vi "Automatic EMS.vi"(8 "error in":errorcluster, 11 "Master Controller in":refnum<class "EMS User Interface.lvclass">) -> (0 "error out":errorcluster, 3 "dup Master Controller out":refnum<class "EMS User Interface.lvclass">)   [LabVIEW 2018, in "EMS User Interface Actor.lvlib" / "EMS User Interface.lvclass"]
uses:
  EMS User Interface.lvclass
  EMS User Interface.lvclass/EMS User Interface.ctl
  <vilib>/ActorFramework/Message Enqueuer/Message Enqueuer.lvclass/Message Enqueuer.ctl
  <vilib>/ActorFramework/Message Enqueuer/Message Priority.ctl
  <vilib>/ActorFramework/Message Enqueuer/Enqueue.vi
  EMS Core/EMS Messages/Stop Init Msg/Stop Init Msg.lvclass
  C:/Program Files (x86)/National Instruments/LabVIEW 2018/vi.lib/ActorFramework/Message/Message.lvclass
  <vilib>/ActorFramework/Message Priority Queue/Priority Enqueue.vi
  <vilib>/ActorFramework/Message Enqueuer/Message Enqueuer.lvclass
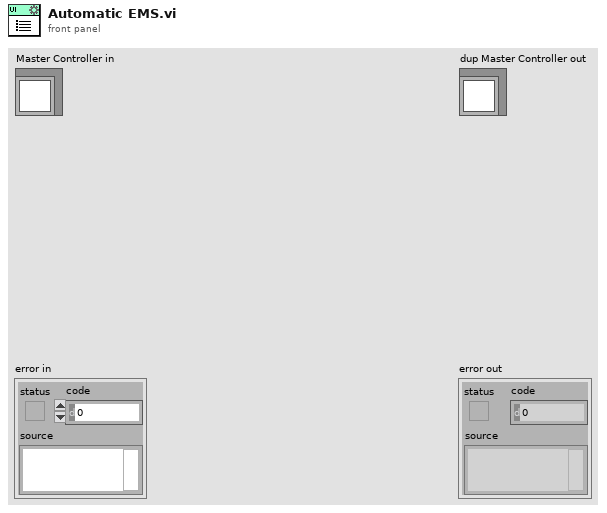
[diagram p1: front panel]
types:
  T1 = typedef "Actor Framework.lvlib/Message Enqueuer.lvclass/Message Priority.ctl" = enum16{"Low", "Normal", "High"}
  T2 = typedef "EMS Core.lvlib/EMS.lvclass/Microgrid State.ctl" = enum16{"Discovery", "Commissioning", "Activation", "Blackstart", "OnGrid", "OffGrid", "Island", "Resynchronization", "Manual", "Shutdown", "Stop"}
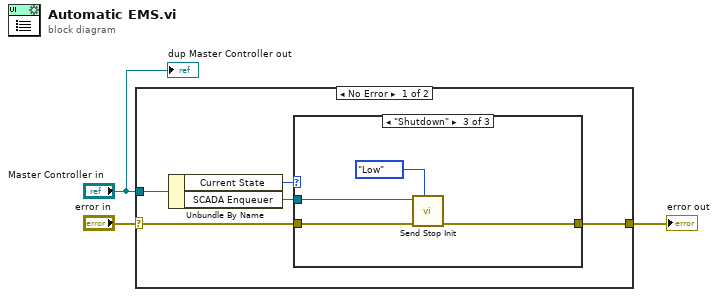
[diagram p0: block diagram]
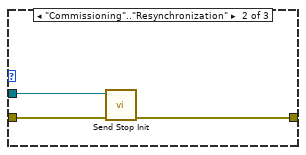
[diagram p3: hidden frame]
diagram:
  n1 = case shown="No Error" "error in" {
    selector: "error in" -> [w7 w17]
    tunnel: [w8 w17] -> w2
    tunnel: "Master Controller in" -> [w5 _]
    frame No Error {
      n2 = Unbundle By Name(w5) -> ("Current State"=w6:T2, "SCADA Enqueuer"=w4:refnum<class "Message Enqueuer.lvclass">)
      n3 = case shown="\"Shutdown\"" w6 {
        tunnel: [w9 w11 w14] -> w8
        tunnel: w7 -> [w9 w12 w16]
        tunnel: w4 -> [_ w10 w15]
        frame "Discovery", Default {
        }
        frame "Commissioning".."Resynchronization" {
          n4 = call "Send Stop Init.vi"("error in (no error)"=w12, "Message Enqueuer"=w10) -> ("error out"=w11:errorcluster)  [unwired: 8 in, 1 out]
        }
        frame "Shutdown" {
          n5 = call "Send Stop Init.vi"("Message Priority (Normal)"=Message_Priority."Low", "error in (no error)"=w16, "Message Enqueuer"=w15) -> ("error out"=w14:errorcluster)  [unwired: 7 in, 1 out]
        }
      }
    }
    frame Error {
    }
  }
  "error out" <- w2
  "dup Master Controller out" <- "Master Controller in"
